vi "c_ctre_phoenix6_platform_write_integer_array.vi"(0 "String 2":string, 1 "Numeric 3":i64, 2 "Numeric 4":u8, 3 "String 4":string, 4 "Numeric 5":dbl) -> (20 "Numeric":i32, 21 "String":string, 22 "Numeric 2":i64, 23 "String 3":string)   [LabVIEW 2023]
uses:
  <vilib>/Rock Robotics/WPI/ThirdParty/Phoenix-LabVIEW/Controls/DriverLib.ctl
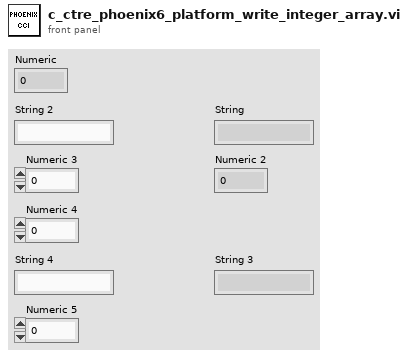
[diagram p1: front panel]
types:
  T1 = typedef "DriverLib.ctl" = path
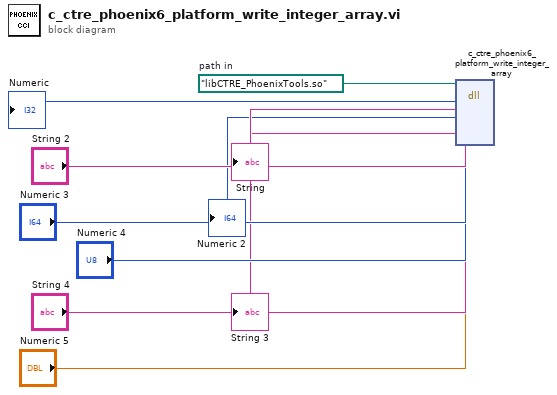
[diagram p0: block diagram]
diagram:
  w10 = T1 path "libCTRE_PhoenixTools.so"  # path in
  n1 = dll-call lib="?" fn="c_ctre_phoenix6_platform_write_integer_array"(path in=w10, "String 2", "Numeric 3", "Numeric 4", "String 4", "Numeric 5") -> (→"Numeric":i32, →"String":string, →"Numeric 2":i64, →"String 3":string)  [unwired: 4 in, 2 out]
